vi "RunInputFile.vi"(9 "Output Path":path, 10 "Input Path":path, 11 "COM Port":refnum<visa-resource-name>) -> ()   [LabVIEW 2010]
uses:
  <vilib>/Utility/file.llb/Read From Spreadsheet File (string).vi
panel:
  out "Array":string[][](array[string])
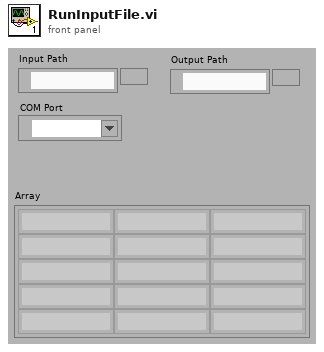
[diagram p1: front panel]
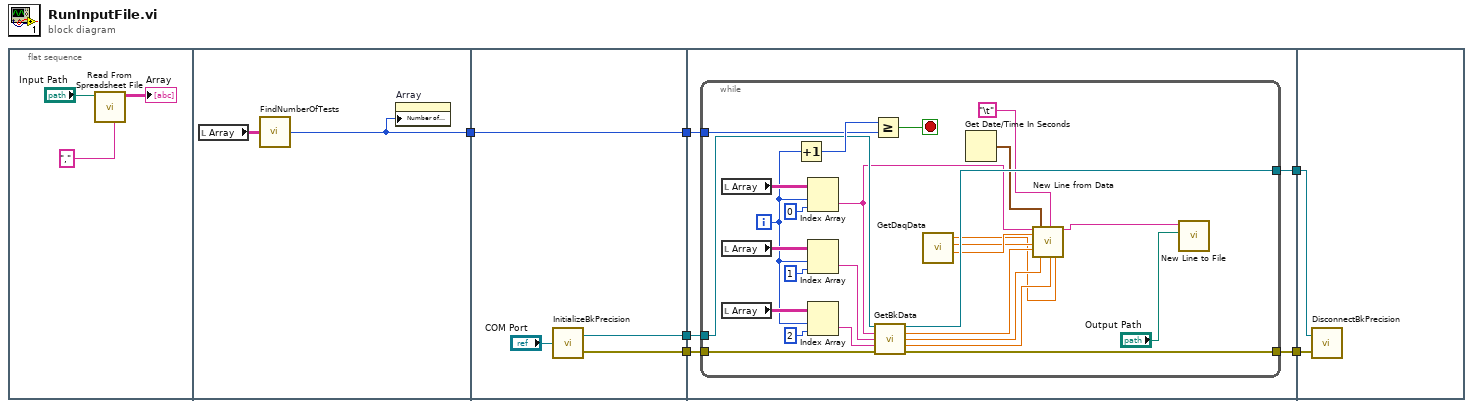
[diagram p0: block diagram]
diagram:
  n1 = flat-sequence {
    tunnel: [w10] -> w3
    tunnel: [w14] -> w6
    tunnel: [w13] -> w5
    tunnel: [w12] -> w4
    tunnel: w3 -> [w12]
    tunnel: w6 -> [w20]
    tunnel: w5 -> [w19]
    tunnel: w4 -> [w18]
    tunnel: [w17] -> w2
    tunnel: [w16] -> w1
    tunnel: w2 -> [w49]
    tunnel: w1 -> [w48]
    frame #0 {
      n2 = call-poly <vilib>:"Read From Spreadsheet File.vi"("delimiter (\\t)"=",", "file path (dialog if empty)"="Input Path") -> ("all rows"=→"Array":string[][])  [unwired: 5 in, 4 out]
    }
    frame #1 {
      n3 = local read "Array"() -> (w11:string[][])
      n4 = call "FindNumberOfTests.vi"("Array"=w11) -> ("Numeric"=w10:i32)
      n5 = property on="Array" class="Arr (strict)"("Number of Rows"=w10) -> ()  [unwired: 2 in, 2 out]
    }
    frame #2 {
      n6 = call "InitializeBkPrecision.vi"("COM Port"="COM Port") -> ("error out"=w13:errorcluster, "VISA resource name out"=w14:refnum<visa-resource-name>)
    }
    frame #3 {
      n7 = while {
        tunnel: w20 -> [w39]
        tunnel: w19 -> [w38]
        tunnel: w18 -> [w41]
        tunnel: [w37] -> w17
        tunnel: [w36] -> w16
        i -> [w33]
        stop <- w43 stop-if-true
        n8 = local read "Array"() -> (w47:string[][])
        n9 = local read "Array"() -> (w46:string[][])
        n10 = local read "Array"() -> (w35:string[][])
        n11 = Increment(x=w33) -> (x+1=w42:i32)
        n12 = Index Array(array=w47, index (row)=w33, index (col)=0) -> (element=w31:string)
        n13 = Index Array(array=w46, index (row)=w33, index (col)=1) -> (element=w40:string)
        n14 = Index Array(array=w35, index (row)=w33, index (col)=2) -> (element=w32:string)
        n15 = Greater Or Equal?(x=w42, y=w41) -> (x >= y?=w43:bool)
        n16 = call "GetBkData.vi"("VISA resource name"=w39, "Mode"=w31, "Value"=w40, "Delay"=w32, "error"=w38) -> ("VISA resource name out"=w37:refnum<visa-resource-name>, "Voltage"=w27:dbl, "Current"=w28:dbl, "Power"=w29:dbl, "error out"=w36:errorcluster)  [unwired: 6 in]
        n17 = call "GetDaqData.vi"() -> ("Amperage across shunt"=w26:dbl, "Light Resistance"=w25:dbl, "Temperature in Celsius"=w24:dbl)  [unwired: 9 in]
        n18 = Get Date/Time In Seconds() -> (seconds since 1Jan1904=w23:timestamp)
        n19 = call "New Line from Data.vi"("Mode"=w31, "DAQ A"=w26, "DAQ R"=w25, "BK V"=w27, "DateTime Stamp"=w23, "BK I"=w28, "Delimiter Character"="\t", "BK P"=w29, "DAQ T"=w24) -> ("String"=w22:string)  [unwired: 10 in]
        n20 = call "New Line to File.vi"("Output File"="Output Path", "Text to add"=w22) -> ()  [unwired: 10 in]
      }
    }
    frame #4 {
      n21 = call "DisconnectBkPrecision.vi"("error out"=w48, "VISA resource name out"=w49) -> ()  [unwired: 1 in]
    }
  }
